vi "Startup.vi"(6 "LabVIEW Web Service":refnum<class "Web Service.lvclass">) -> ()   [LabVIEW 2015]
uses:
  <vilib>/wsapi/Web Service.lvclass
  GlobalSender.vi
panel:
  # "Use the web service input terminal to call the VIs on the Service subpalette of the Web Services palette. Do not remove it from the connector pane unless you don't need access to the palette."
  # "Any additional terminals added to the connector pane of a startup VI will be ignored."
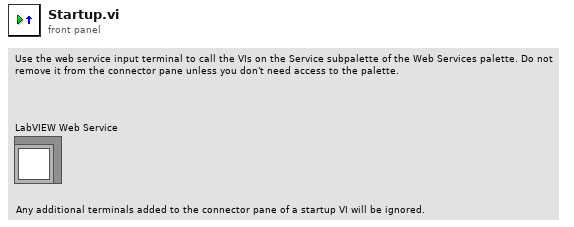
[diagram p1: front panel]
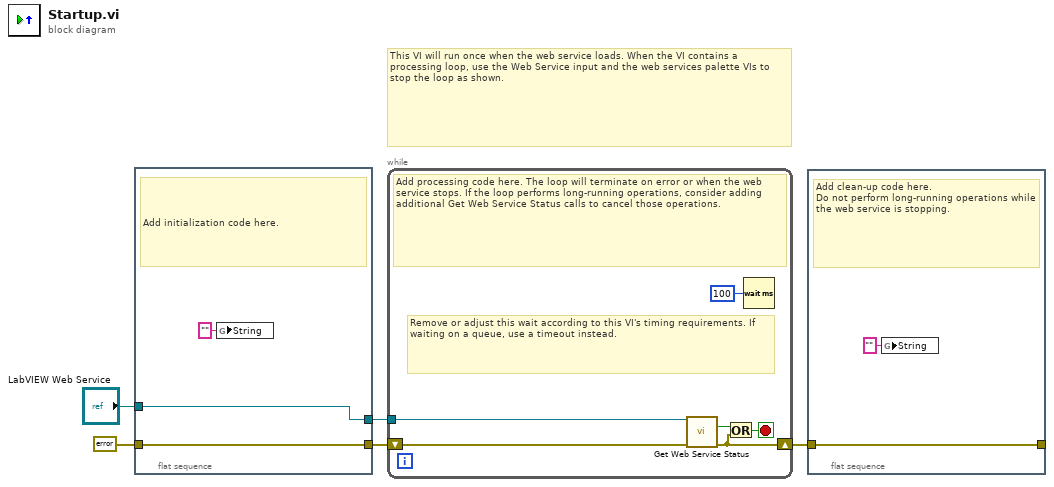
[diagram p0: block diagram]
diagram:
  # "This VI will run once when the web service loads. When the VI contains a processing loop, use the Web Service input and the web services palette VIs to stop the loop as shown."
  n1 = flat-sequence {
    tunnel: "LabVIEW Web Service" -> [w8]
    tunnel: [w8] -> w4
    tunnel: [w7] -> w3
    tunnel: errorcluster {"status"=FALSE, "code"=0, "source"=""} ("error constant") -> [w7]
    frame #0 {
      # "Add initialization code here."
      n2 = global write "GlobalSender.vi" "String"("" ("String")) -> ()
    }
  }
  n3 = while {
    tunnel: w4 -> [w13]
    shift-right: [w10] -> w1
    shift-left: w3 -> [w11]
    stop <- w12 stop-if-true
    # "Remove or adjust this wait according to this VI's timing requirements. If waiting on a queue, use a timeout instead."
    # "Add processing code here. The loop will terminate on error or when the web service stops. If the loop performs long-running operations, consider adding additional Get Web Service Status calls to cancel those operations."
    n4 = call <vilib>:"Get Web Service Status.vi"("LabVIEW Web Service"=w13, "error in (no error)"=w11) -> ("service stopping?"=w14:bool, "error out"=w10:errorcluster)  [unwired: 11 in, 1 out]
    n5 = Or(x=w14, y=w10) -> (x .or. y?=w12:bool)
    n6 = Wait (ms)(milliseconds to wait=u32 100) -> ()  [unwired: 1 out]
  }
  n7 = flat-sequence {
    tunnel: [w16] -> _
    tunnel: w1 -> [w16]
    frame #0 {
      # "Add clean-up code here.\nDo not perform long-running operations while the web service is stopping."
      n8 = global write "GlobalSender.vi" "String"("" ("String")) -> ()
    }
  }
